vi "Handle Notification.vi"(8 "error in (no error)":errorcluster, 9 "Payload":string, 10 "Notification Type":string, 11 "Test Sequencer in":refnum<class "Sequencer with Output Values.lvclass">) -> (0 "error out":errorcluster, 3 "Test Sequencer out":refnum<class "Sequencer with Output Values.lvclass">)   [LabVIEW 2020, in "Sequencer with Output Values.lvlib" / "Sequencer with Output Values.lvclass"]
uses:
  Sequencer with Output Values.lvclass
  Sequencer with Output Values.lvclass/Sequencer with Output Values.ctl
  Global Strings.vi
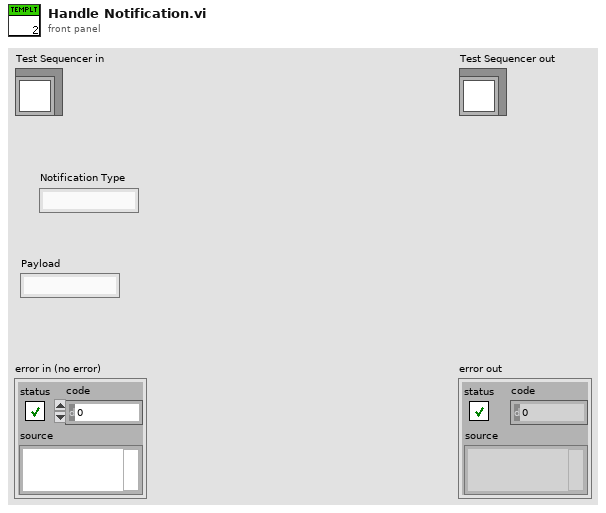
[diagram p1: front panel]
types:
  T1 = typedef "Sequencer with Output Values.lvlib/Sequencer with Output Values.lvclass/Params.ctl" = cluster{"Step Values":T2[], "Only Execute When Test Running":bool, "Current Sequence ID":u32, "Total Iterations":u32, "Last Timestamp":timestamp, "Number of Sequence Steps":i32, "Number of Analog Channels":i32, "Number of Digital Channels":i32, "Delay Before Starting Sequence":dbl}
  T2 = typedef "Step Settings.ctl" = cluster{"Duration":dbl, "Mode":string, "Delay Between Values":dbl, "Analog Values":string[], "Digital Values":string[]}
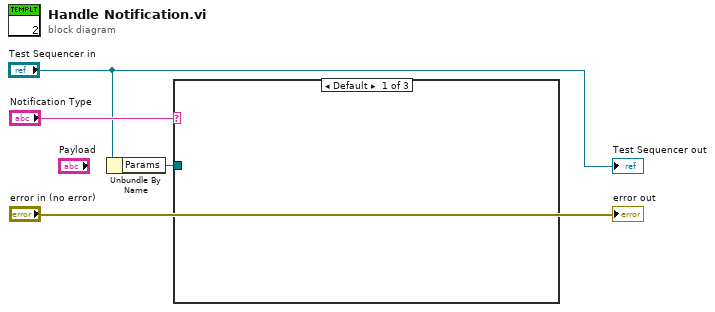
[diagram p0: block diagram]
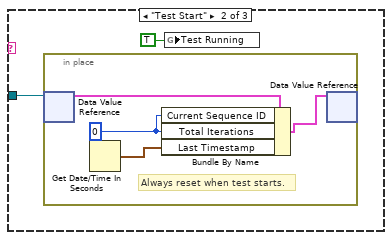
[diagram p2: hidden frame]
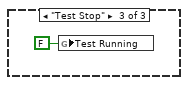
[diagram p3: hidden frame]
diagram:
  n1 = Unbundle By Name("Test Sequencer in") -> ("Params"=w1:refnum<data-value>)
  n2 = case shown="Default" "Notification Type" {
    tunnel: w1 -> [_ w6 _]
    frame Default {
    }
    frame "Test Start" {
      n3 = in-place {
        w8 = u32 0 ("Total Iterations")
        # "Always reset when test starts."
        n4 = in-place-dvr #1(w6) -> (w10:T1)  [unwired: 1 out]
        n5 = Get Date/Time In Seconds ("t0")() -> (seconds since 1Jan1904=w7:timestamp)
        n6 = Bundle By Name(cluster=w10, "Current Sequence ID"=w8, "Total Iterations"=w8, "Last Timestamp"=w7) -> (w9:T1)
        n7 = in-place-dvr #1(w9) -> ()  [unwired: 2 out]
      }
      n8 = global write "Global Strings.vi" "Test Running"(TRUE ("Test Running")) -> ()
    }
    frame "Test Stop" {
      n9 = global write "Global Strings.vi" "Test Running"(FALSE ("Test Running")) -> ()
    }
  }
  "error out" <- "error in (no error)"
  "Test Sequencer out" <- "Test Sequencer in"
